vi "add_CMDState.vi"(6 "State":T1, 7 "msg in":string) -> (3 "msg out":string)   [LabVIEW 2018]
doc: "Flattens a pose 2D into a message"
uses:
  <userlib>/ROS for LabVIEW Software/ROS/MessageBuilding/std_msgs/subs/float64Scalar.vi
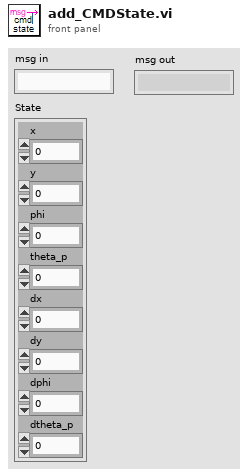
[diagram p1: front panel]
types:
  T1 = cluster{"x":dbl, "y":dbl, "phi":dbl, "theta_p":dbl, "dx":dbl, "dy":dbl, "dphi":dbl, "dtheta_p":dbl}
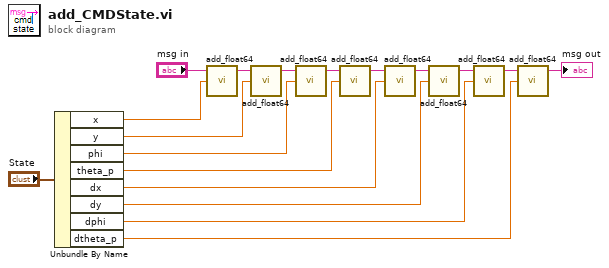
[diagram p0: block diagram]
diagram:
  n1 = Unbundle By Name("State") -> ("x"=w10:dbl, "y"=w9:dbl, "phi"=w8:dbl, "theta_p"=w7:dbl, "dx"=w6:dbl, "dy"=w5:dbl, "dphi"=w4:dbl, "dtheta_p"=w1:dbl)
  n2 = call-poly <userlib>:"add_float64.vi"("Numeric"=w10, "msg in"="msg in") -> ("msg out"=w16:string)  [unwired: 3 in]
  n3 = call-poly <userlib>:"add_float64.vi"("Numeric"=w9, "msg in"=w16) -> ("msg out"=w15:string)  [unwired: 3 in]
  n4 = call-poly <userlib>:"add_float64.vi"("Numeric"=w8, "msg in"=w15) -> ("msg out"=w14:string)  [unwired: 3 in]
  n5 = call-poly <userlib>:"add_float64.vi"("Numeric"=w7, "msg in"=w14) -> ("msg out"=w13:string)  [unwired: 3 in]
  n6 = call-poly <userlib>:"add_float64.vi"("Numeric"=w6, "msg in"=w13) -> ("msg out"=w12:string)  [unwired: 3 in]
  n7 = call-poly <userlib>:"add_float64.vi"("Numeric"=w5, "msg in"=w12) -> ("msg out"=w11:string)  [unwired: 3 in]
  n8 = call-poly <userlib>:"add_float64.vi"("Numeric"=w4, "msg in"=w11) -> ("msg out"=w2:string)  [unwired: 3 in]
  n9 = call-poly <userlib>:"add_float64.vi"("Numeric"=w1, "msg in"=w2) -> ("msg out"=→"msg out":string)  [unwired: 3 in]
